vi "Tools_Windows Get Locale.vi"(8 "error in (no error)":errorcluster) -> (0 "error out":errorcluster, 1 "Locale RegKey (Hex)":string, 3 "Locale":T1)   [LabVIEW 2014]
uses:
  <vilib>/registry/registry.llb/Registry RtKey.ctl
  <vilib>/registry/registry.llb/Read Registry Value Simple STR.vi
  tools_windows Locales.ctl
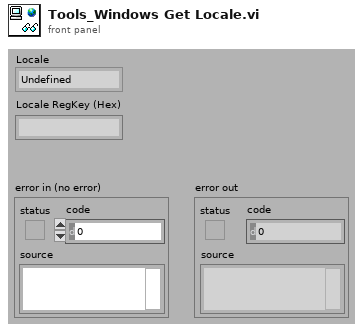
[diagram p1: front panel]
types:
  T1 = typedef "tools_windows Locales.ctl" = enum16{"Undefined", "English (US)", "French", "Spanish", "Portugese", "German", "Korean", "Chinese (Simplified)", "Chinese (Traditional)", "Japanese"}
  T2 = typedef "Registry RtKey.ctl" = enum32{"HKEY_CLASSES_ROOT", "HKEY_CURRENT_USER", "HKEY_LOCAL_MACHINE", "HKEY_USERS", "HKEY_PERFORMANCE_DATA", "HKEY_CURRENT_CONFIG", "HKEY_DYN_DATA"}
  T3 = typedef "Registry refnum.ctl" = refnum<k1>
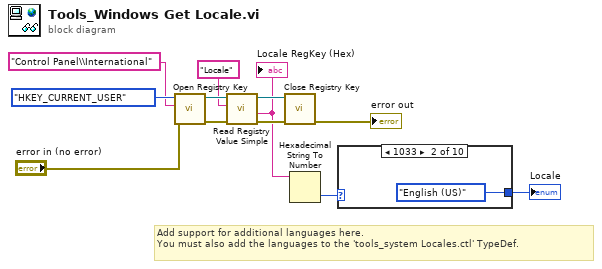
[diagram p0: block diagram]
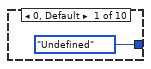
[diagram p2: hidden frame]
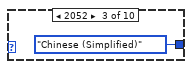
[diagram p3: hidden frame]
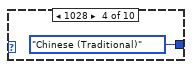
[diagram p4: hidden frame]
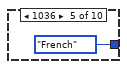
[diagram p5: hidden frame]
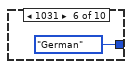
[diagram p6: hidden frame]
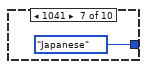
[diagram p7: hidden frame]
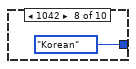
[diagram p8: hidden frame]
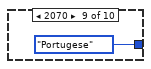
[diagram p9: hidden frame]
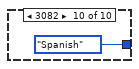
[diagram p10: hidden frame]
diagram:
  # "Add support for additional languages here.\nYou must also add the languages to the 'tools_system Locales.ctl' TypeDef."
  n1 = call <vilib>:"Open Registry Key.vi"("error in (no error)"="error in (no error)", "subkey"="Control Panel\\International", "root key (HKEY_LOCAL_MACHINE)"=Registry_RtKey."HKEY_CURRENT_USER") -> ("error out"=w11:errorcluster, "refnum out"=w10:T3)  [unwired: 7 in]
  n2 = call-poly <vilib>:"Read Registry Value Simple.vi"("error in (no error)"=w11, "value"="Locale", "refnum"=w10) -> ("error out"=w9:errorcluster, "String/Binary data"=w6:string, "refnum out"=w8:T3)  [unwired: 3 in, 1 out]
  "Locale RegKey (Hex)" <- w6
  n3 = call <vilib>:"Close Registry Key.vi"("error in (no error)"=w9, "refnum"=w8) -> ("error out"=→"error out":errorcluster)  [unwired: 5 in]
  n4 = Hexadecimal String To Number(string=w6) -> (number=w5:u32)  [unwired: 2 in, 1 out]
  n5 = case shown="1033" w5 {
    tunnel: [tools_windows_Locales."Undefined" ("Locale") tools_windows_Locales."English (US)" ("Locale") tools_windows_Locales."Chinese (Simplified)" ("Locale") tools_windows_Locales."Chinese (Traditional)" ("Locale") tools_windows_Locales."French" ("Locale") tools_windows_Locales."German" ("Locale") tools_windows_Locales."Japanese" ("Locale") tools_windows_Locales."Korean" ("Locale") tools_windows_Locales."Portugese" ("Locale") tools_windows_Locales."Spanish" ("Locale")] -> w4
    frame 0, Default {
    }
    frame 1033 {
    }
    frame 2052 {
    }
    frame 1028 {
    }
    frame 1036 {
    }
    frame 1031 {
    }
    frame 1041 {
    }
    frame 1042 {
    }
    frame 2070 {
    }
    frame 3082 {
    }
  }
  "Locale" <- w4
